vi "Get Active Window_KT.vi"() -> (2 "Name":string, 3 "hWnd":u32)   [LabVIEW 2017, in "KTools.lvlib"]
doc: "<------Get Active Window------>\nReturns handle & name of the active window."
uses:
  KTools.lvlib
  user32.dll
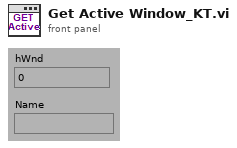
[diagram p1: front panel]
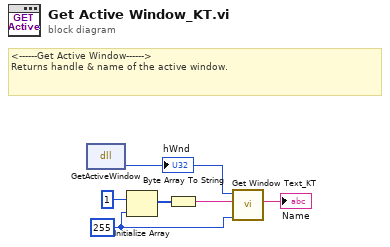
[diagram p0: block diagram]
diagram:
  w2 = 255 ("dimension size")
  # "<------Get Active Window------>\nReturns handle & name of the active window."
  n1 = dll-call lib="user32.dll" fn="GetActiveWindow"() -> ("hWnd"=w6:u32)  [unwired: 3 in, 2 out]
  "hWnd" <- w6
  n2 = Initialize Array(1 ("uCmd"), w2) -> (w5:i32[])
  n3 = Byte Array To String(unsigned byte array=w5) -> (string=w3:string)
  n4 = call "Get Window Text_KT.vi"("nMaxCount"=w2, "Name (Byte)"=w3, "hWnd"=w6) -> ("Name"=→"Name":string)  [unwired: 5 in, 1 out]
